vi "Speech Recognizer Initialize.vi"(9 "String[] phrases":string[](array[string]), 10 "Score":refnum<vi>, 11 "Text":refnum<vi>) -> (0 "error out":errorcluster, 2 "Event Callback":refnum<k27>, 3 "reference":refnum<k24>)   [LabVIEW 2017]
uses:
  System.Speech
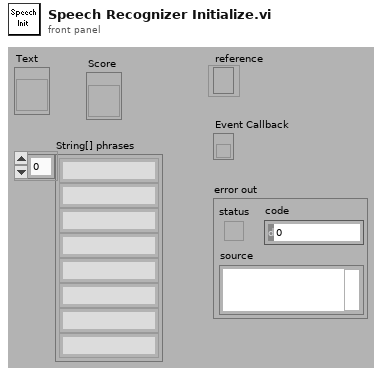
[diagram p1: front panel]
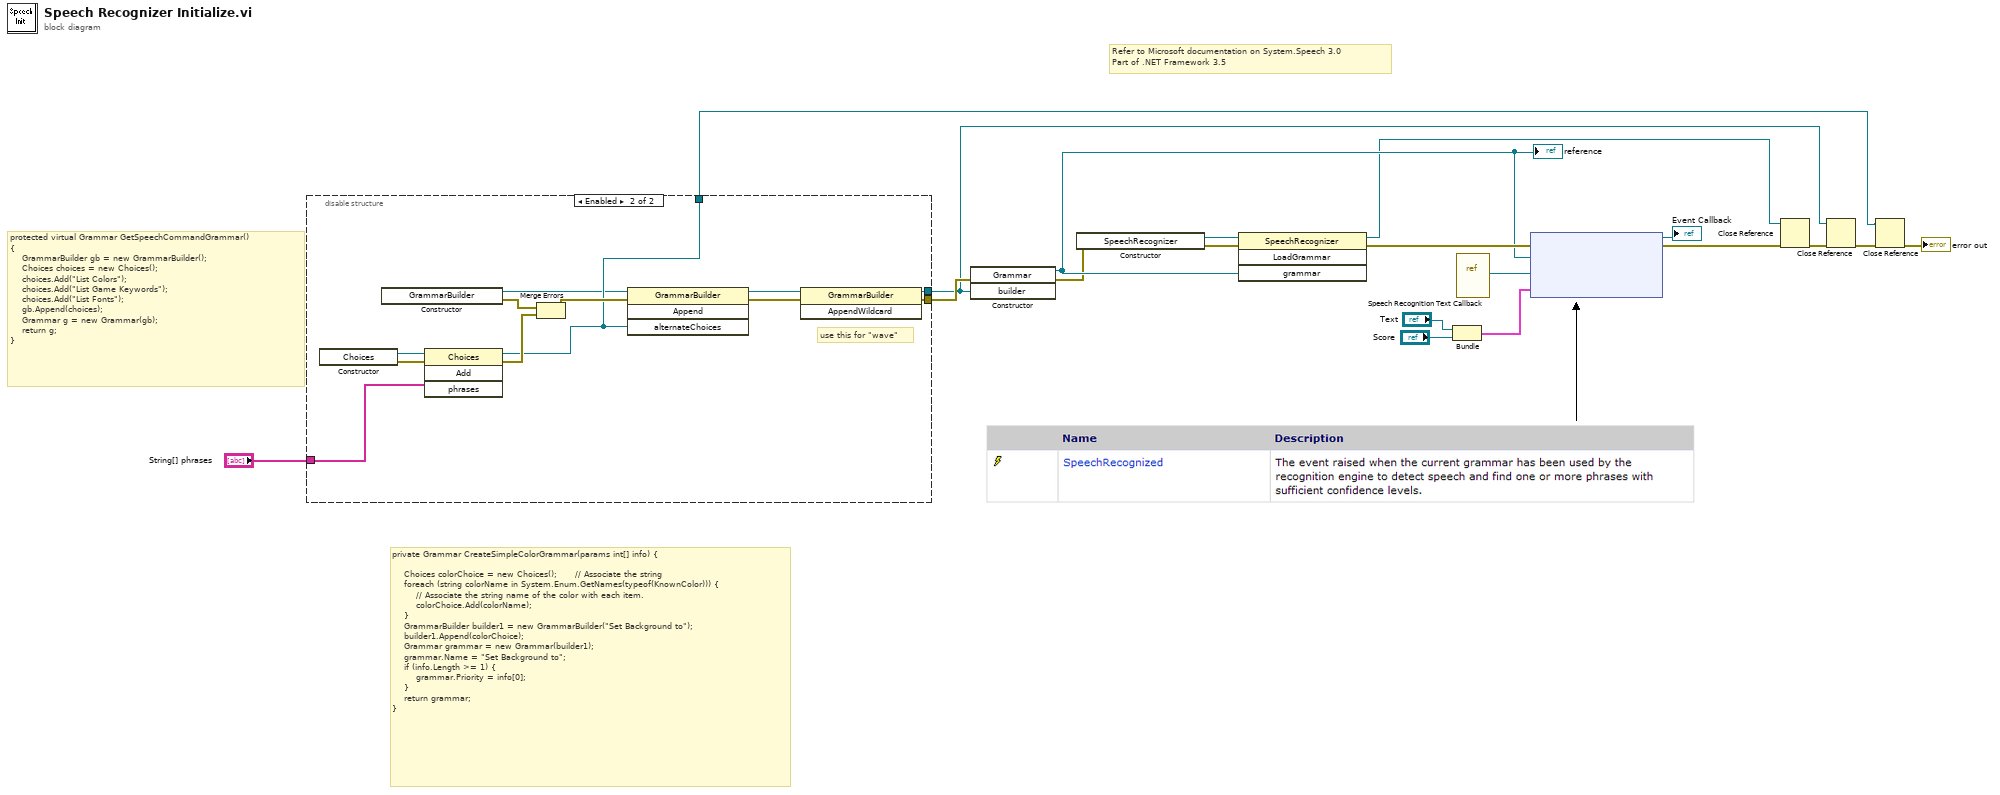
[diagram p0: block diagram]
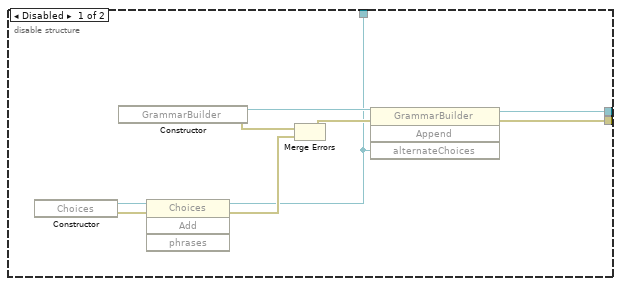
[diagram p2: hidden frame]
diagram:
  # "private Grammar CreateSimpleColorGrammar(params int[] info) {\n    \n    Choices colorChoice = new Choices();      // Associate the string \n    foreach (string colorName in System.Enum.GetNames(typeof(KnownColor))) {\n        // Associate the string name of the color with each item.\n        colorChoice.Add(colorName);\n    }\n    GrammarBuilder builder1 = new GrammarBuilder(\"Set Background to\");\n    builder1.Append(colorChoice);\n    Grammar grammar = new Grammar(builder1);\n    grammar.Name = \"Set Background to\";\n    if (info.Length >= 1) {\n        grammar.Priority = info[0];\n    }\n    return grammar;\n}"
  # "protected virtual Grammar GetSpeechCommandGrammar()\n{\n    GrammarBuilder gb = new GrammarBuilder();\n    Choices choices = new Choices();\n    choices.Add(\"List Colors\");\n    choices.Add(\"List Game Keywords\");\n    choices.Add(\"List Fonts\");\n    gb.Append(choices);\n    Grammar g = new Grammar(gb);\n    return g;\n}"
  # "Refer to Microsoft documentation on System.Speech 3.0\nPart of .NET Framework 3.5"
  n1 = disable-structure shown="Enabled" {
    disable-tunnel: [w26 w34] -> w7
    disable-tunnel: [w22 w35] -> w6
    disable-tunnel: [w21 w33] -> w5
    disable-tunnel: "String[] phrases" -> [_ w30]
    frame Disabled {
      n2 = constructor class="Choices"() -> (reference out=w29:refnum<k24>, error out=w28:errorcluster)  [unwired: 3 in, 1 out]
      n3 = constructor class="GrammarBuilder"() -> (reference out=w27:refnum<k24>, error out=w24:errorcluster)  [unwired: 3 in, 1 out]
      n4 = invoke class="Choices" method="Add"(reference=w29, error in=w28) -> (reference out=w21:refnum<k24>, error out=w25:errorcluster, "phrases"=w20:string[])  [unwired: 1 in, 2 out]
      n5 = Merge Errors(w24, w25) -> (w23:errorcluster)
      n6 = invoke class="GrammarBuilder" method="Append"(reference=w27, error in=w23, "alternateChoices"=w21) -> (reference out=w22:refnum<k24>, error out=w26:errorcluster)  [unwired: 1 in, 2 out]
    }
    frame Enabled {
      # "use this for \"wave\""
      n7 = constructor class="Choices"() -> (reference out=w36:refnum<k24>, error out=w41:errorcluster)  [unwired: 3 in, 1 out]
      n8 = constructor class="GrammarBuilder"() -> (reference out=w31:refnum<k24>, error out=w39:errorcluster)  [unwired: 3 in, 1 out]
      n9 = invoke class="Choices" method="Add"(reference=w36, error in=w41, "phrases"=w30) -> (reference out=w33:refnum<k24>, error out=w38:errorcluster)  [unwired: 1 in, 2 out]
      n10 = Merge Errors(w39, w38) -> (w40:errorcluster)
      n11 = invoke class="GrammarBuilder" method="Append"(reference=w31, error in=w40, "alternateChoices"=w33) -> (reference out=w37:refnum<k24>, error out=w32:errorcluster)  [unwired: 1 in, 2 out]
      n12 = invoke class="GrammarBuilder" method="AppendWildcard"(reference=w37, error in=w32) -> (reference out=w35:refnum<k24>, error out=w34:errorcluster)  [unwired: 1 in, 1 out]
    }
  }
  n13 = constructor class="Grammar"(error in=w7, "builder"=w6) -> (reference out=w8:refnum<k24>, error out=w4:errorcluster)  [unwired: 2 in, 2 out]
  "reference" <- w8
  n14 = constructor class="SpeechRecognizer"(error in=w4) -> (reference out=w15:refnum<k24>, error out=w16:errorcluster)  [unwired: 2 in, 1 out]
  n15 = invoke class="SpeechRecognizer" method="LoadGrammar"(reference=w15, error in=w16, "grammar"=w8) -> (reference out=w2:refnum<k24>, error out=w14:errorcluster)  [unwired: 1 in, 2 out]
  n16 = Bundle("Text"="Text", "Score"="Score") -> (w3:cluster{"Text":refnum<vi>, "Score":refnum<vi>})  [unwired: 1 out]
  n17 = vi-ref "Speech Recognition Text Callback.vi"() -> (w9:refnum<vi>)
  n18 = node(w14, w8, w9, w3) -> (→"Event Callback":refnum<k27>, w13:errorcluster)  [unwired: 1 in]
  n19 = Close Reference(reference=w2, error in (no error)=w13) -> (error out=w19:errorcluster)
  n20 = Close Reference(reference=w6, error in (no error)=w19) -> (error out=w18:errorcluster)
  n21 = Close Reference(reference=w5, error in (no error)=w18) -> (error out=→"error out":errorcluster)
